vi "write_jt_headers_to_data_file.vi"(11 "file path in":path) -> (3 "file path out":path)   [LabVIEW 2016]
uses:
  <vilib>/Utility/file.llb/Write Delimited Spreadsheet (string).vi
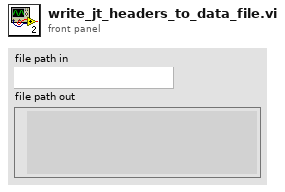
[diagram p1: front panel]
types:
  T1 = enum16{"open", "replace", "create", "open or create", "replace or create", "replace or create with confirmation"}
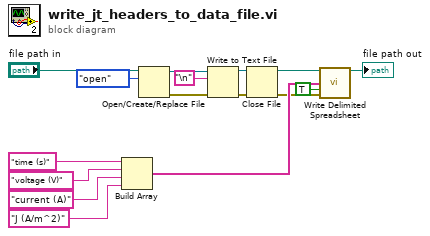
[diagram p0: block diagram]
diagram:
  n1 = Build Array("time (s)", "voltage (V)", "current (A)", "J (A/m^2)") -> (w11:string[])
  n2 = Open/Create/Replace File(file path (use dialog)="file path in", operation (0:open)=T1."open") -> (refnum out=w7:refnum<file>, error out=w6:errorcluster)  [unwired: 4 in, 1 out]
  n3 = Write to Text File(file (use dialog)=w7, text="\n", error in=w6) -> (refnum out=w5:refnum<file>, error out=w4:errorcluster)  [unwired: 1 in, 1 out]
  n4 = Close File(refnum=w5, error in=w4) -> (path=w3:path, error out=w2:errorcluster)
  n5 = call-poly <vilib>:"Write Delimited Spreadsheet.vi"("file path (dialog if empty)"=w3, "1D data"=w11, "append to file? (new file:F)"=TRUE, "error in (no error)"=w2) -> ("new file path (Not A Path if cancelled)"=→"file path out":path)  [unwired: 10 in, 1 out]
